vi "calibrate DO.vi"(11 "Index":u32) -> ()   [LabVIEW 2015]
uses:
  toolbar icons/help.ctl
  TCP DAQ/zero.ctl
  DAQ configuration/Sensor buffer command.ctl
  <vilib>/Platform/browser.llb/Open URL in Default Browser (string).vi
panel:
  out "Saturated voltage":dbl format="%.3f"
  in  "Zero":T1
  in  "Help Button":T2
  in  "local atm":bool
  out "Sample Temperature":dbl[unit] format="%.1f"
  in  "Set to Saturated Do":bool
  in  "OK Button":bool
  out "name":string
  out "units":string
  in  "Temperature\nChannel":i32 min=0 step=1
  in  "Temperature\ncompensated":bool
  in  "Barometric pressure":dbl[unit]=101300.0
  out "DO":dbl[unit] format="%.1f"
  out "DO voltage":dbl[unit] format="%.1f"
  out "XY Graph":cluster{dbl[], dbl[]}[](graph)
  out "Quit":bool
  in  "Temperature":sgl[unit]=293.15 format="%.2f"
  out "DO sat (mg/L)":dbl format="%.2f"
  # "zero in oxygen free water (do this first)"
  # "in saturated water"
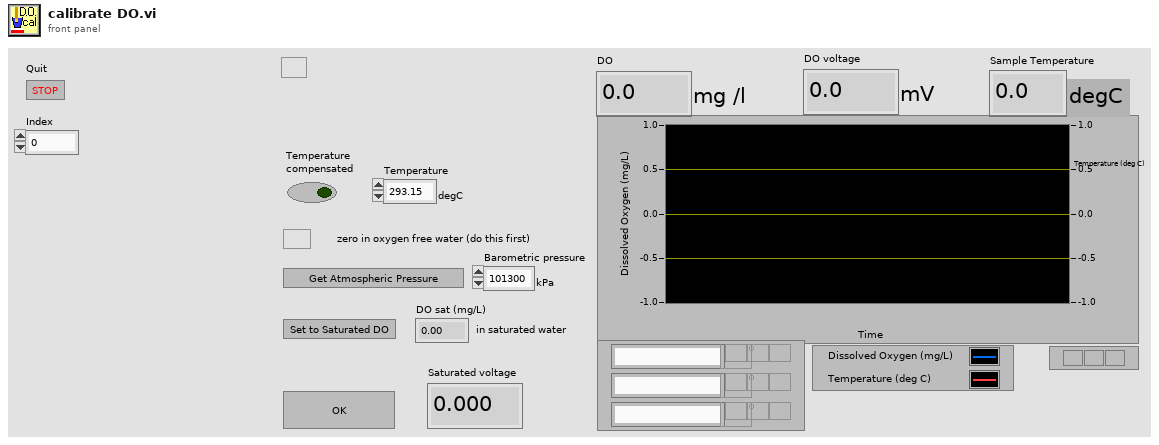
[diagram p1: front panel]
types:
  T1 = typedef "zero.ctl" = bool
  T2 = typedef "help.ctl" = bool
  T3 = typedef "Sensor buffer command.ctl" = enum16{"read average", "read recent", "read all", "write", "set buffer size", "Read channel config", "Write channel config", "clear"}
  T4 = enum16{"Volts", "Polynomial", "Correspondence Table", "pH", "Dissolved Oxygen"}
  T5 = typedef "Channel config.ctl" = cluster{"Channel Indices":T6[], "AI Max voltage":dbl[], "Calibration matrix":T7}
  T6 = typedef "channel identifier.ctl" = u16
  T7 = typedef "calib array.ctl" = T8[]
  T8 = typedef "conversion.ctl" = cluster{"conversion matrix":sgl[][], "units":string, "name":string, "scale type":T9, "offset (volts)":dbl, "second channel":i8, "correspondence table":T10, "offset (physical units)":dbl, "pH scale":T11, "D.O.":T12, "Photometer data":T13}
  T9 = typedef "scale type.ctl" = enum16{"Volts", "Polynomial", "Correspondence Table", "pH", "Dissolved Oxygen", "Quadratic", "Photometer"}
  T10 = typedef "correspondence table.ctl" = cluster{"physical units":dbl, "volts":dbl}[]
  T11 = typedef "pH scale.ctl" = cluster{"Buffers":cluster{"Buffer":dbl, "Calibrated":bool, "V/T":dbl}[], "Temperature":dbl}
  T12 = typedef "DO scale.ctl" = cluster{"Temperature":dbl, "K":dbl, "barometric pressure":dbl}
  T13 = typedef "Photometer calibration data.ctl" = cluster{"Dark Voltage":dbl, "Blank Voltage":dbl, "Standards":cluster{"Concentration":dbl, "Voltage":dbl}[]}
  T14 = typedef "Sensor data.ctl" = cluster{" Sensor array":T15[], "Time":dbl}
  T15 = typedef "sensor cluster.ctl" = cluster{"voltage":sgl, "scaled":sgl, "units":string, "Out of Range":bool}
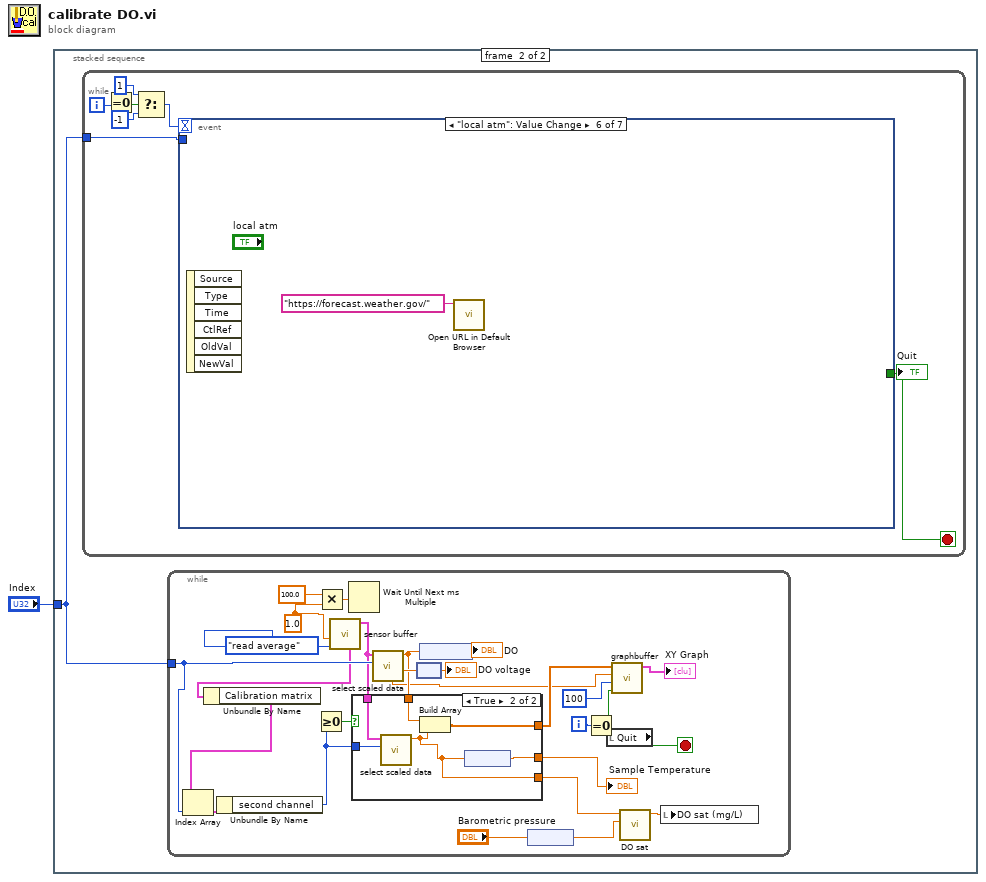
[diagram p0: block diagram]
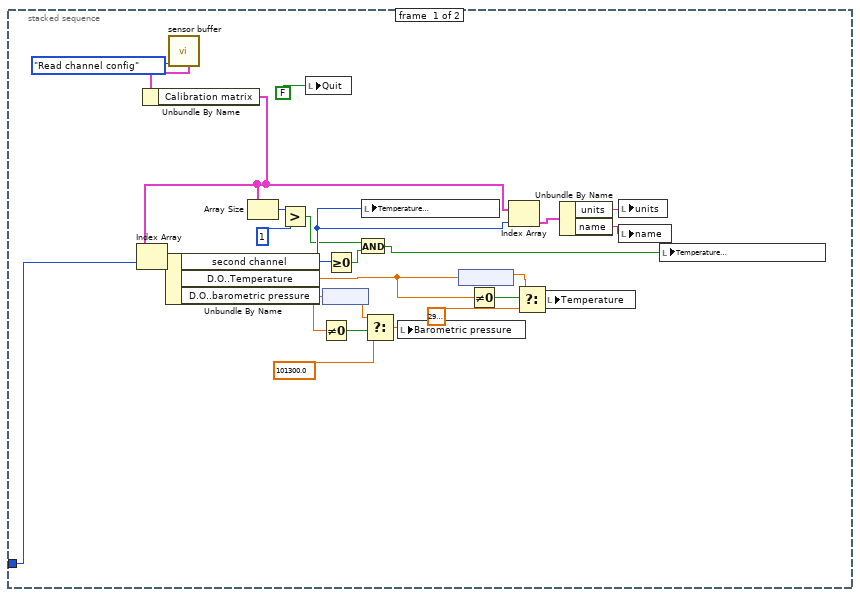
[diagram p2: hidden frame]
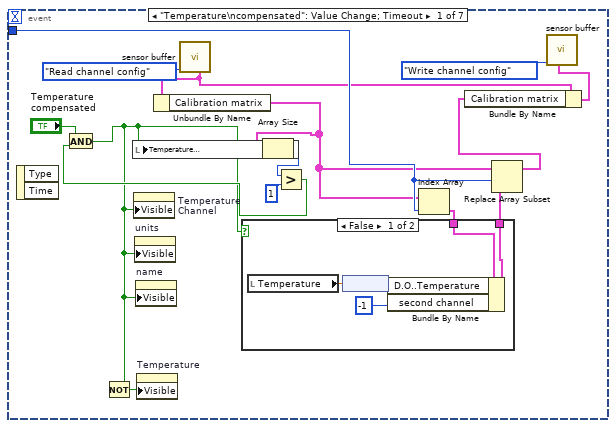
[diagram p3: hidden frame]
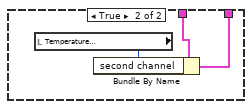
[diagram p4: hidden frame]
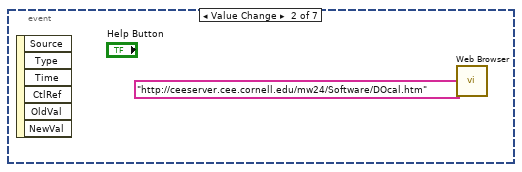
[diagram p5: hidden frame]
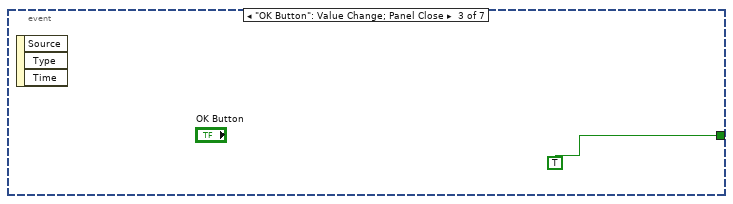
[diagram p6: hidden frame]
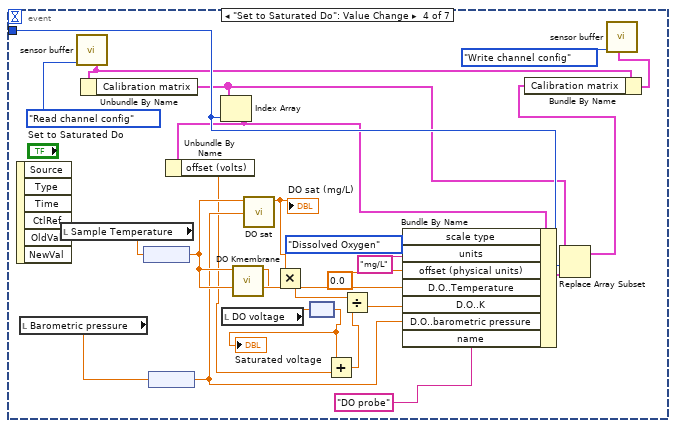
[diagram p7: hidden frame]
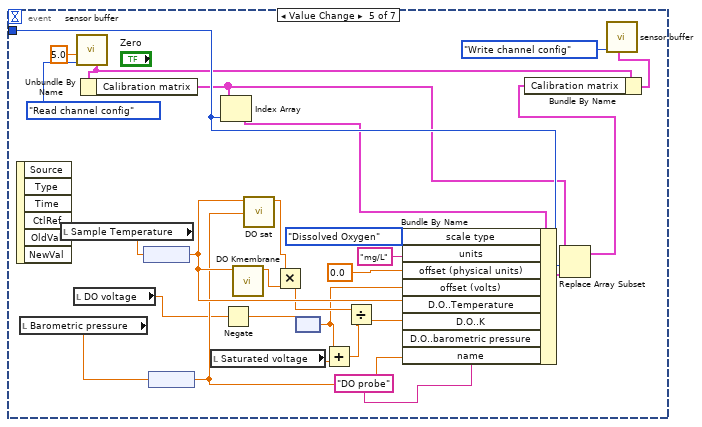
[diagram p8: hidden frame]
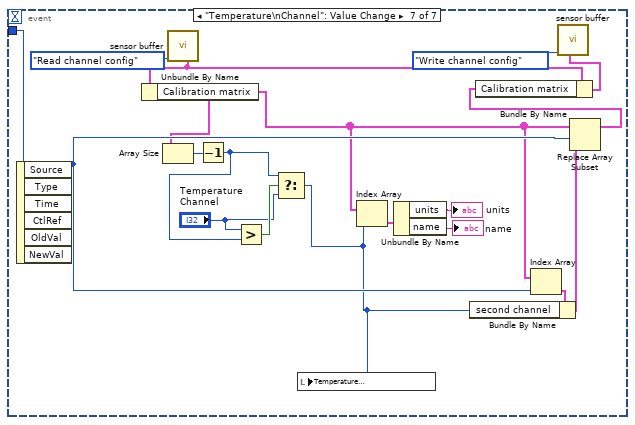
[diagram p9: hidden frame]
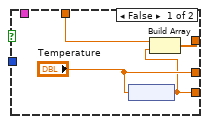
[diagram p10: hidden frame]
diagram:
  n1 = stacked-sequence {
    tunnel: "Index" -> [w24 w27]
    frame #0 {
      n2 = call "sensor buffer.vi"("command"=Sensor_buffer_command."Read channel config") -> ("Channel Config out"=w4:T5)  [unwired: 6 in, 4 out]
      n3 = Unbundle By Name(w4) -> ("Calibration matrix"=w2:T7)
      n4 = Index Array(array=w2, index=w24) -> (element=w26:T8)
      n5 = Unbundle By Name(w26) -> ("second channel"=w21:i8, "D.O..Temperature"=w15:dbl, "D.O..barometric pressure"=w17:dbl)
      n6 = Array Size(array=w2) -> (size(s)=w10:i32)
      n7 = Greater?(x=w10, y=1) -> (0:w8:bool)
      n8 = local write "Quit"(FALSE ("Quit")) -> ()
      n9 = Not Equal To 0?(x=w17) -> (x != 0?=w16:bool)
      n10 = node(w17) -> (w18:dbl[unit])
      n11 = Greater Or Equal To 0?(x=w21) -> (x >= 0?=w7:bool)
      n12 = And(x=w8, y=w7) -> (x .and. y?=w6:bool)
      n13 = local write "Temperature\nChannel"(w21) -> ()
      n14 = Select(t=w18, s=w16, f=dbl[unit] 101300.0) -> (s? t:f=w19:dbl[unit])
      n15 = local write "Barometric pressure"(w19) -> ()
      n16 = node(w15) -> (w14:dbl[unit])
      n17 = Not Equal To 0?(x=w15) -> (x != 0?=w12:bool)
      n18 = Index Array(array=w2, index=w21) -> (element=w25:T8)
      n19 = Select(t=w14, s=w12, f=dbl[unit] 295.15) -> (s? t:f=w13:dbl[unit])
      n20 = local write "Temperature"(w13) -> ()
      n21 = Unbundle By Name(w25) -> ("units"=w22:string, "name"=w23:string)
      n22 = local write "units"(w22) -> ()
      n23 = local write "name"(w23) -> ()
      n24 = local write "Temperature\ncompensated"(w6) -> ()
    }
    frame #1 {
      n25 = while {
        tunnel: w27 -> [w34]
        i -> [w29]
        stop <- w33 stop-if-true
        n26 = Equal To 0?(x=w29) -> (x = 0?=w28:bool)
        n27 = Select(t=1, s=w28, f=-1) -> (s? t:f=w32:i32)
        n28 = event shown="[5] \"local atm\": Value Change" {
          selector: _ -> [_ _ _ _ _ _ _]
          dyn-events: _ -> [_ _ _ _ _ _ _]
          timeout: w32 -> [_ _ _ _ _ _ _]
          tunnel: w34 -> [w47 _ _ w73 w100 _ w124]
          tunnel: [_ _ TRUE ("OK Button") _ _ _ _] -> w33
          event "Temperature\ncompensated": Value Change; Timeout {
            n29 = event-data() -> ()  [unwired: 1 in, 2 out]
            n30 = call "sensor buffer.vi"("command"=Sensor_buffer_command."Read channel config") -> ("Channel Config out"=w37:T5)  [unwired: 6 in, 4 out]
            n31 = Unbundle By Name(w37) -> ("Calibration matrix"=w39:T7)
            n32 = Array Size(array=w39) -> (size(s)=w45:i32)
            n33 = Greater?(x=w45, y=1) -> (0:w43:bool)
            n34 = And(x="Temperature\ncompensated", y=w43) -> (x .and. y?=w41:bool)
            n35 = Not(x=w41) -> (.not. x?=w46:bool)
            n36 = local write "Temperature\ncompensated"(w41) -> ()
            n37 = property on="Temperature\nChannel" class="DigNum (strict)"("Visible"=w41) -> ()  [unwired: 2 in, 2 out]
            n38 = property on="units" class="Str"("Visible"=w41) -> ()  [unwired: 2 in, 2 out]
            n39 = property on="name" class="Str"("Visible"=w41) -> ()  [unwired: 2 in, 2 out]
            n40 = property on="Temperature" class="DigNum (strict)"("Visible"=w46) -> ()  [unwired: 2 in, 2 out]
            n41 = Index Array(array=w39, index=w47) -> (element=w49:T8)
            n42 = case shown="False" w41 {
              tunnel: w49 -> [w54 w56]
              tunnel: [w53 w55] -> w48
              frame False {
                n43 = local read "Temperature"() -> (w51:sgl[unit])
                n44 = node(w51) -> (w50:sgl)
                n45 = Bundle By Name(cluster=w54, "D.O..Temperature"=w50, "second channel"=i8 -1) -> (w53:T8)
              }
              frame True {
                n46 = local read "Temperature\nChannel"() -> (w57:i32)
                n47 = Bundle By Name(cluster=w56, "second channel"=w57) -> (w55:T8)
              }
            }
            n48 = Replace Array Subset(array=w39, new element=w48, index=w47) -> (w36:T7)
            n49 = Bundle By Name(cluster=w37, "Calibration matrix"=w36) -> (w35:T5)
            n50 = call "sensor buffer.vi"("Channel Config"=w35, "command"=Sensor_buffer_command."Write channel config") -> ()  [unwired: 5 in, 5 out]
          }
          event Value Change {
            n51 = event-data() -> ()  [unwired: 1 in, 6 out]
            n52 = call "Web Browser.vi"("URL"="http://ceeserver.cee.cornell.edu/mw24/Software/DOcal.htm") -> ()  [unwired: 1 in]
          }
          event "OK Button": Value Change; Panel Close {
            n53 = event-data() -> ()  [unwired: 1 in, 3 out]
          }
          event "Set to Saturated Do": Value Change {
            n54 = event-data() -> ()  [unwired: 1 in, 6 out]
            n55 = local read "Barometric pressure"() -> (w82:dbl[unit])
            n56 = local read "Sample Temperature"() -> (w83:dbl[unit])
            n57 = call "sensor buffer.vi"("command"=Sensor_buffer_command."Read channel config") -> ("Channel Config out"=w68:T5)  [unwired: 6 in, 4 out]
            n58 = Unbundle By Name(w68) -> ("Calibration matrix"=w70:T7)
            n59 = node(w83) -> (w84:dbl)
            n60 = node(w82) -> (w72:dbl)
            n61 = Index Array(array=w70, index=w73) -> (element=w64:T8)
            n62 = Unbundle By Name(w64) -> ("offset (volts)"=w63:dbl)
            n63 = local read "DO voltage"() -> (w61:dbl[unit])
            n64 = call "DO Kmembrane.vi"("Temperature (C)"=w84) -> ("Kmembrane"=w74:dbl)  [unwired: 10 in]
            n65 = call "DO sat.vi"("Atmospheric Pressure (kPa)"=w72, "Temperature (C)"=w84) -> ("DO sat (mg/L)"=w76:dbl)  [unwired: 9 in]
            "DO sat (mg/L)" <- w76
            n66 = Multiply(x=w76, y=w74) -> (x*y=w75:dbl)
            n67 = node(w61) -> (w60:dbl)
            "Saturated voltage" <- w60
            n68 = Add(x=w60, y=w63) -> (x+y=w62:dbl)
            n69 = Divide(x=w75, y=w62) -> (x/y=w80:dbl)
            n70 = Bundle By Name(cluster=w64, "scale type"=T4."Dissolved Oxygen", "units"="mg/L", "offset (physical units)"=0.0, "D.O..Temperature"=w84, "D.O..K"=w80, "D.O..barometric pressure"=w72, "name"="DO probe") -> (w81:T8)
            n71 = Replace Array Subset(array=w70, new element=w81, index=w73) -> (w67:T7)
            n72 = Bundle By Name(cluster=w68, "Calibration matrix"=w67) -> (w66:T5)
            n73 = call "sensor buffer.vi"("Channel Config"=w66, "command"=Sensor_buffer_command."Write channel config") -> ()  [unwired: 5 in, 5 out]
          }
          event Value Change {
            n74 = event-data() -> ()  [unwired: 1 in, 6 out]
            n75 = local read "Barometric pressure"() -> (w109:dbl[unit])
            n76 = local read "Sample Temperature"() -> (w110:dbl[unit])
            n77 = local read "DO voltage"() -> (w89:dbl[unit])
            n78 = call "sensor buffer.vi"("command"=Sensor_buffer_command."Read channel config", "smooth interval (s)"=sgl 5.0) -> ("Channel Config out"=w95:T5)  [unwired: 5 in, 4 out]
            n79 = Unbundle By Name(w95) -> ("Calibration matrix"=w97:T7)
            n80 = node(w110) -> (w111:dbl)
            n81 = node(w109) -> (w99:dbl)
            n82 = local read "Saturated voltage"() -> (w88:dbl)
            n83 = Index Array(array=w97, index=w100) -> (element=w91:T8)
            n84 = Negate(x=w89) -> (-x=w85:dbl[unit])
            n85 = call "DO Kmembrane.vi"("Temperature (C)"=w111) -> ("Kmembrane"=w101:dbl)  [unwired: 10 in]
            n86 = call "DO sat.vi"("Atmospheric Pressure (kPa)"=w99, "Temperature (C)"=w111) -> ("DO sat (mg/L)"=w103:dbl)  [unwired: 9 in]
            n87 = Multiply(x=w103, y=w101) -> (x*y=w102:dbl)
            n88 = node(w85) -> (w87:dbl)
            n89 = Add(x=w87, y=w88) -> (x+y=w90:dbl)
            n90 = Divide(x=w102, y=w90) -> (x/y=w107:dbl)
            n91 = Bundle By Name(cluster=w91, "scale type"=T4."Dissolved Oxygen", "units"="mg/L", "offset (physical units)"=0.0, "offset (volts)"=w87, "D.O..Temperature"=w111, "D.O..K"=w107, "D.O..barometric pressure"=w99, "name"="DO probe") -> (w108:T8)
            n92 = Replace Array Subset(array=w97, new element=w108, index=w100) -> (w94:T7)
            n93 = Bundle By Name(cluster=w95, "Calibration matrix"=w94) -> (w93:T5)
            n94 = call "sensor buffer.vi"("Channel Config"=w93, "command"=Sensor_buffer_command."Write channel config") -> ()  [unwired: 5 in, 5 out]
          }
          event "local atm": Value Change {
            n95 = event-data() -> ()  [unwired: 1 in, 6 out]
            n96 = call-poly <vilib>:"Open URL in Default Browser.vi"("URL"="https://forecast.weather.gov/") -> ()  [unwired: 5 in, 2 out]
          }
          event "Temperature\nChannel": Value Change {
            n97 = event-data() -> ()  [unwired: 1 in, 6 out]
            n98 = call "sensor buffer.vi"("command"=Sensor_buffer_command."Read channel config") -> ("Channel Config out"=w115:T5)  [unwired: 6 in, 4 out]
            n99 = Unbundle By Name(w115) -> ("Calibration matrix"=w117:T7)
            n100 = Array Size(array=w117) -> (size(s)=w123:i32)
            n101 = Decrement(x=w123) -> (x-1=w121:i32)
            n102 = Greater?(x="Temperature\nChannel", y=w121) -> (0:w122:bool)
            n103 = Select(t=w121, s=w122, f="Temperature\nChannel") -> (s? t:f=w119:i32)
            n104 = local write "Temperature\nChannel"(w119) -> ()
            n105 = Index Array(array=w117, index=w119) -> (element=w129:T8)
            n106 = Unbundle By Name(w129) -> ("units"=→"units":string, "name"=→"name":string)
            n107 = Index Array(array=w117, index=w124) -> (element=w128:T8)
            n108 = Bundle By Name(cluster=w128, "second channel"=w119) -> (w127:T8)
            n109 = Replace Array Subset(array=w117, new element=w127, index=w124) -> (w114:T7)
            n110 = Bundle By Name(cluster=w115, "Calibration matrix"=w114) -> (w113:T5)
            n111 = call "sensor buffer.vi"("Channel Config"=w113, "command"=Sensor_buffer_command."Write channel config") -> ()  [unwired: 5 in, 5 out]
          }
        }
        "Quit" <- w33
      }
      n112 = while {
        tunnel: w27 -> [w143]
        i -> [w152]
        stop <- w156 stop-if-true
        w133 = sgl 1.0 ("smooth interval (s)")
        n113 = Multiply(x=100.0 ("y"), y=w133) -> (x*y=w155:dbl)
        n114 = call "sensor buffer.vi"("command"=Sensor_buffer_command."read average", "smooth interval (s)"=w133) -> ("Calibrated data"=w134:T14, "Channel Config out"=w132:T5)  [unwired: 5 in, 3 out]
        n115 = Unbundle By Name(w132) -> ("Calibration matrix"=w131:T7)
        n116 = Index Array(array=w131, index=w143) -> (element=w147:T8)
        n117 = Unbundle By Name(w147) -> ("second channel"=w146:i8)
        n118 = Greater Or Equal To 0?(x=w146) -> (x >= 0?=w145:bool)
        n119 = Wait Until Next ms Multiple(millisecond multiple=w155) -> ()  [unwired: 1 out]
        n120 = call "select scaled data.vi"("Sensor index"=w143, "Sensor Data"=w134) -> ("voltage"=w148:sgl, "scaled"=w142:sgl, "Time"=w130:dbl)  [unwired: 4 in, 3 out]
        n121 = case shown="True" w145 {
          tunnel: w134 -> [_ w166]
          tunnel: w146 -> [_ w165]
          tunnel: w142 -> [w160 w164]
          tunnel: [w159 w163] -> w144
          tunnel: ["Temperature" w162] -> w139
          tunnel: [w157 w161] -> w138
          frame False {
            n122 = node("Temperature") -> (w157:sgl)
            n123 = Build Array(w160, w157) -> (w159:sgl[])
          }
          frame True {
            n124 = call "select scaled data.vi"("Sensor index"=w165, "Sensor Data"=w166) -> ("scaled"=w161:sgl)  [unwired: 4 in, 5 out]
            n125 = Build Array(w164, w161) -> (w163:sgl[])
            n126 = node(w161) -> (w162:sgl[unit])
          }
        }
        "Sample Temperature" <- w139
        n127 = node(w148) -> (→"DO voltage":sgl[unit])
        n128 = node(w142) -> (→"DO":sgl[unit])
        n129 = node("Barometric pressure") -> (w136:dbl)
        n130 = Equal To 0?(x=w152) -> (x = 0?=w151:bool)
        n131 = local read "Quit"() -> (w156:bool)
        n132 = call "graphbuffer.vi"("Reset"=w151, "history length"=u16 100, "Time"=w130, "data"=w144) -> ("Multiplot graph data"=→"XY Graph":cluster{dbl[], dbl[]}[])  [unwired: 5 in, 2 out]
        n133 = call "DO sat.vi"("Atmospheric Pressure (kPa)"=w136, "Temperature (C)"=w138) -> ("DO sat (mg/L)"=w140:dbl)  [unwired: 9 in]
        n134 = local write "DO sat (mg/L)"(w140) -> ()
      }
    }
  }
